vi "move.vi"(0 "M1 Info in":cluster{"M1 distance":dbl, "velocityM1":dbl}, 1 "M2 Info in":cluster{"M2 distance":dbl, "velocityM2":dbl}, 2 "button com":bool, 3 "max 1":dbl, 4 "max 2":dbl, 5 "handle":i32, 6 "halt":refnum<vi>, 7 "device ID":refnum<k1>, 8 "M3 Info in":cluster{"M3 distance":dbl, "velocityM3":dbl}, 9 "M3 Axis":u16(ring)=5 items=["X axis", "Y axis", "Z axis", "X axis rotation", "Y axis rotation", "Z axis rotation", "U axis", "V axis"], 10 "M1 Axis":u16(ring)=2 items=["X axis", "Y axis", "Z axis", "X axis rotation", "Y axis rotation", "Z axis rotation", "U axis", "V axis"], 11 "M2 Axis":u16(ring)=5 items=["X axis", "Y axis", "Z axis", "X axis rotation", "Y axis rotation", "Z axis rotation", "U axis", "V axis"], 12 "Invert":bool, 13 "Invert 2":bool=TRUE, 18 "Invert 3":bool=TRUE, 19 "max 3":dbl) -> ()   [LabVIEW 2012]
uses:
  <vilib>/Utility/inputDevices.llb/joystickAcquire.vi
  MicroDrive.dll
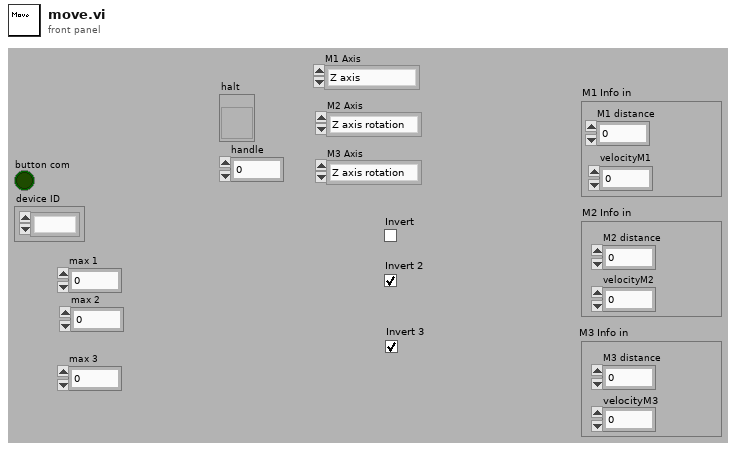
[diagram p1: front panel]
types:
  T1 = cluster{"Boolean array[0]":bool, "Boolean array[1]":bool, "Boolean array[2]":bool, "Boolean array[3]":bool, "Boolean array[4]":bool, "Boolean array[5]":bool, "Boolean array[6]":bool, "Boolean array[7]":bool, "Boolean array[8]":bool, "Boolean array[9]":bool, "Boolean array[10]":bool, "Boolean array[11]":bool, "Boolean array[12]":bool, "Boolean array[13]":bool, "Boolean array[14]":bool, "Boolean array[15]":bool}
  T2 = cluster{"X axis":i32, "Y axis":i32, "Z axis":i32, "X axis rotation":i32, "Y axis rotation":i32, "Z axis rotation":i32, "U axis":i32, "V axis":i32}
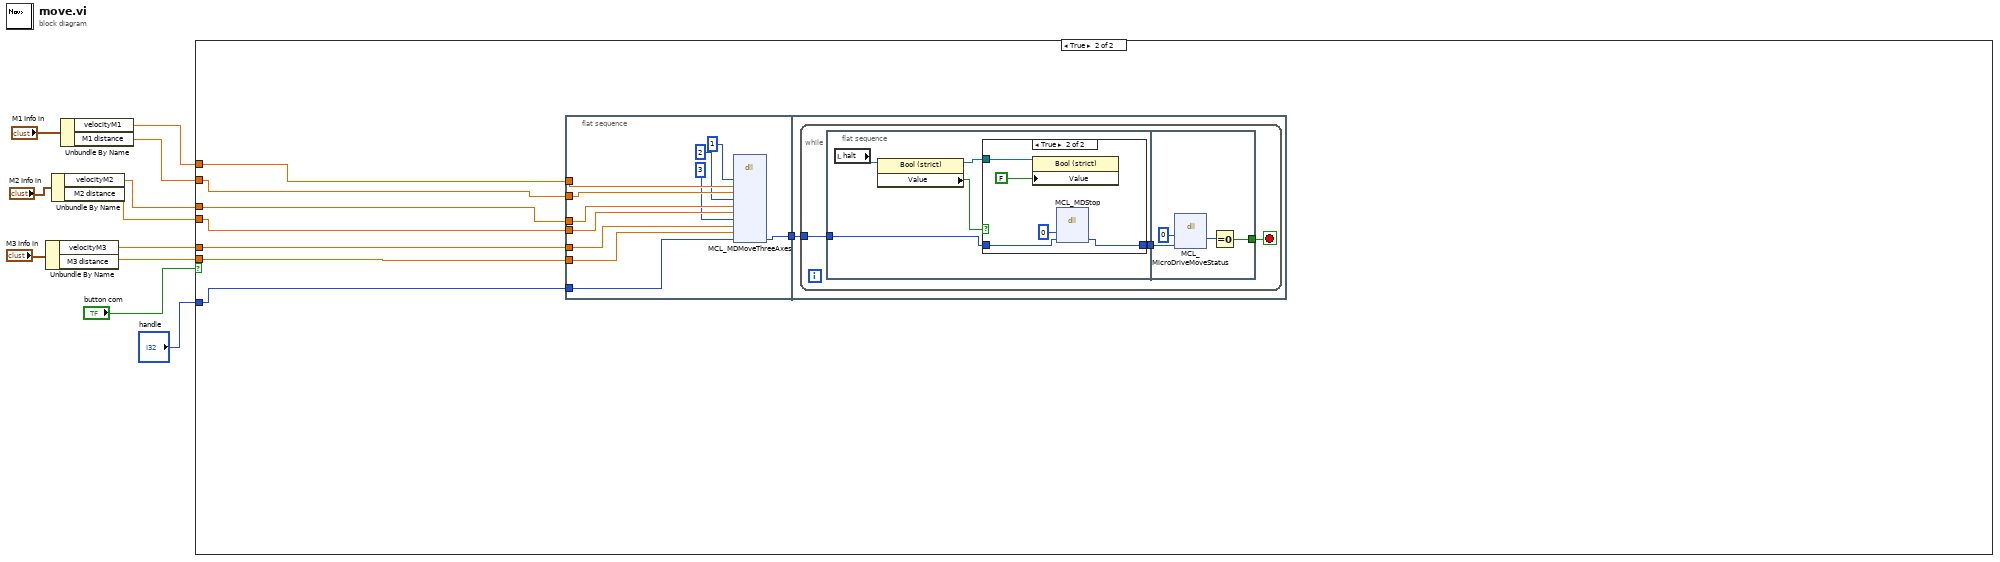
[diagram p0: block diagram]
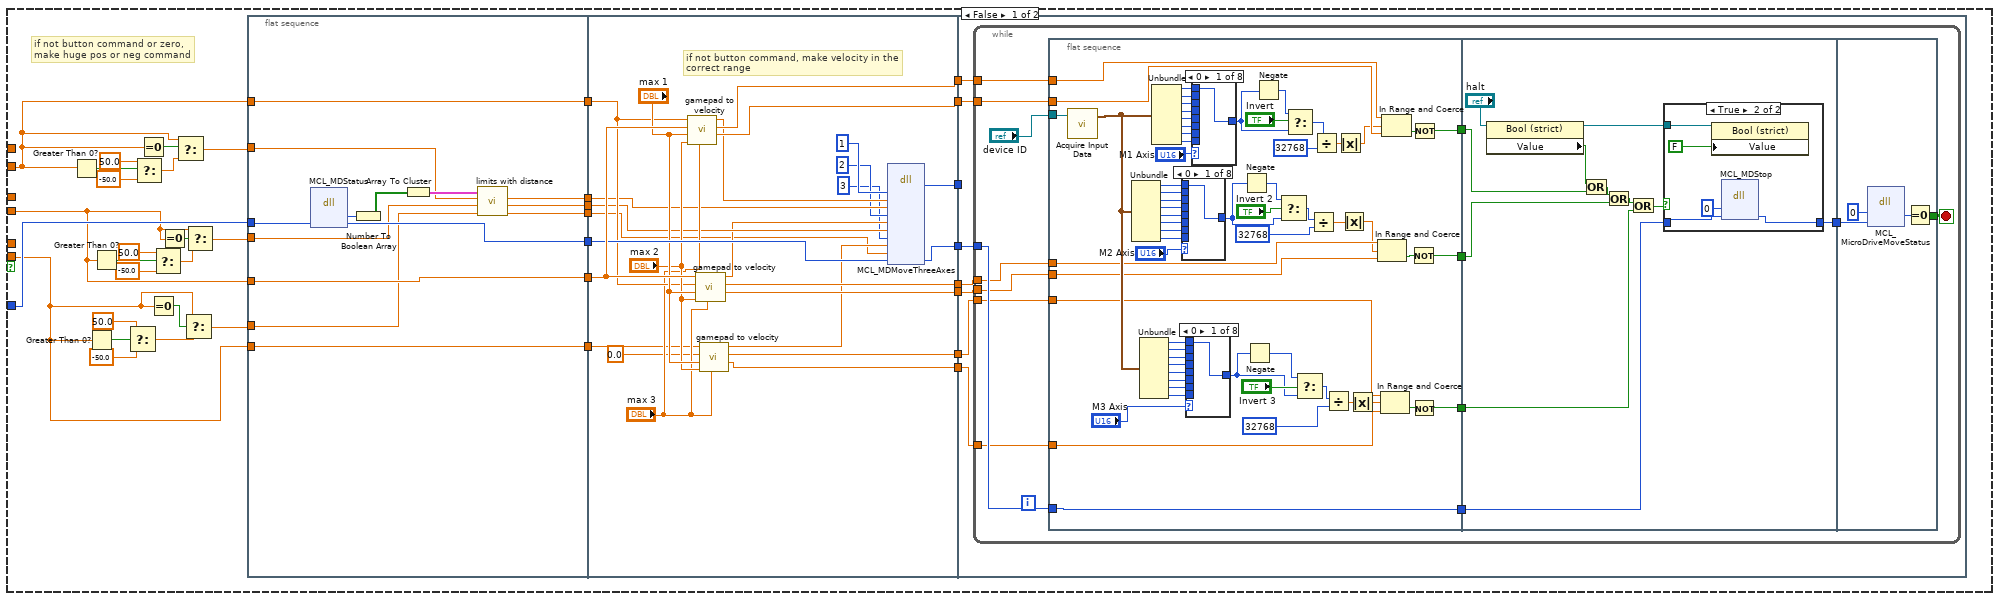
[diagram p2: hidden frame]
diagram:
  n1 = Unbundle By Name("M3 Info in") -> ("velocityM3"=w2:dbl, "M3 distance"=w1:dbl)
  n2 = Unbundle By Name("M2 Info in") -> ("velocityM2"=w4:dbl, "M2 distance"=w5:dbl)
  n3 = Unbundle By Name("M1 Info in") -> ("velocityM1"=w8:dbl, "M1 distance"=w9:dbl)
  n4 = case shown="True" "button com" {
    tunnel: "handle" -> [w29 w224]
    tunnel: w9 -> [w24 w222]
    tunnel: w8 -> [_ w221]
    tunnel: w5 -> [w20 w220]
    tunnel: w4 -> [_ w219]
    tunnel: w2 -> [_ w218]
    tunnel: w1 -> [w13 w217]
    frame False {
      # "if not button command or zero,\nmake huge pos or neg command"
      n5 = Greater Than 0?(x=w24) -> (x > 0?=w39:bool)
      n6 = Greater Than 0?(x=w13) -> (x > 0?=w19:bool)
      n7 = Greater Than 0?(x=w20) -> (x > 0?=w34:bool)
      n8 = Select(t=50.0, s=w19, f=-50.0) -> (s? t:f=w16:dbl)
      n9 = Select(t=50.0, s=w39, f=-50.0) -> (s? t:f=w40:dbl)
      n10 = Equal To 0?(x=w24) -> (x = 0?=w41:bool)
      n11 = Equal To 0?(x=w13) -> (x = 0?=w15:bool)
      n12 = Select(t=50.0, s=w34, f=-50.0) -> (s? t:f=w35:dbl)
      n13 = Equal To 0?(x=w20) -> (x = 0?=w36:bool)
      n14 = Select(t=w24, s=w41, f=w40) -> (s? t:f=w31:dbl)
      n15 = Select(t=w13, s=w15, f=w16) -> (s? t:f=w14:dbl)
      n16 = Select(t=w20, s=w36, f=w35) -> (s? t:f=w30:dbl)
      n17 = flat-sequence {
        tunnel: [w59] -> w48
        tunnel: [w52] -> w47
        tunnel: [w51] -> w46
        tunnel: [w55] -> w45
        tunnel: [w54] -> w44
        tunnel: w29 -> [w60]
        tunnel: w31 -> [w57]
        tunnel: w30 -> [w56]
        tunnel: w24 -> [w55]
        tunnel: w20 -> [w54]
        tunnel: w13 -> [w53]
        tunnel: [w53] -> w21
        tunnel: w14 -> [w50]
        tunnel: [w49] -> w12
        tunnel: [w87] -> w43
        tunnel: w48 -> [w80]
        tunnel: w47 -> [w74]
        tunnel: w46 -> [w73]
        tunnel: w45 -> [w76]
        tunnel: w44 -> [w81]
        tunnel: [w86] -> w42
        tunnel: [w85] -> w28
        tunnel: [w84] -> w27
        tunnel: [w83] -> w26
        tunnel: [w82] -> w25
        tunnel: [w72] -> w23
        tunnel: [w79] -> w22
        tunnel: w21 -> [w70]
        tunnel: w12 -> [w63]
        tunnel: w43 -> [w94]
        tunnel: w42 -> [_]
        tunnel: w28 -> [w93]
        tunnel: w27 -> [w92]
        tunnel: w26 -> [w91]
        tunnel: w25 -> [w90]
        tunnel: w23 -> [w89]
        tunnel: w22 -> [w88]
        frame #0 {
          n18 = dll-call lib="C:/Users/Labview/Desktop/SRR/MicroDrive_x64/Labview Examples/MicroDrive.dll" fn="MCL_MDStatus"("handle"=w60) -> ("status"=w62:u16, "handle"=w59:i32)  [unwired: 3 in, 4 out]
          n19 = Number To Boolean Array(number=w62) -> (Boolean array=w61:bool[])
          n20 = Array To Cluster(array=w61) -> (cluster=w58:T1)
          n21 = call "limits with distance.vi"("distanceM3"=w50, "distanceM2"=w56, "distanceM1"=w57, "cluster"=w58) -> ("M3 Distance"=w49:dbl, "M2 Distance"=w51:dbl, "M1 Distance"=w52:dbl)  [unwired: 5 out]
        }
        frame #1 {
          # "if not button command, make velocity in the\ncorrect range"
          n22 = call "gamepad to velocity.vi"("max 3 axis"="max 3", "max 2 axis"="max 2", "max 1 axis"="max 1", "joystick sub"=w81, "joystick main"=w76) -> ("lower bound"=w84:dbl, "upper bound"=w85:dbl, "Velocity"=w69:dbl)  [unwired: 4 out]
          n23 = call "gamepad to velocity.vi"("max 3 axis"="max 3", "max 2 axis"="max 2", "max 1 axis"="max 1", "joystick sub"=w76, "joystick main"=w81) -> ("lower bound"=w82:dbl, "upper bound"=w83:dbl, "Velocity"=w68:dbl)  [unwired: 4 out]
          n24 = call "gamepad to velocity.vi"("max 3 axis"="max 3", "max 2 axis"="max 2", "max 1 axis"="max 1", "joystick sub"=0.0, "joystick main"=w70) -> ("lower bound"=w79:dbl, "upper bound"=w72:dbl, "Velocity"=w67:dbl)  [unwired: 4 out]
          n25 = dll-call lib="C:/Users/Labview/Desktop/SRR/MicroDrive_x64/Labview Examples/MicroDrive.dll" fn="MCL_MDMoveThreeAxes"("axis1"=1 ("roundingX"), "velocity1"=w69, "distance1"=w74, "axis2"=2 ("roundingX"), "velocity2"=w68, "distance2"=w73, "axis3"=3 ("roundingX"), "velocity3"=w67, "distance3"=w63, "handle"=w80) -> ("return type"=w86:i32, "handle"=w87:i32)  [unwired: 11 in, 3 out]
        }
        frame #2 {
          n26 = while {
            tunnel: w94 -> [w108]
            tunnel: w93 -> [w104]
            tunnel: w92 -> [w103]
            tunnel: w91 -> [w102]
            tunnel: w90 -> [w101]
            tunnel: w89 -> [w97]
            tunnel: w88 -> [w96]
            stop <- w107 stop-if-true
            n27 = flat-sequence {
              tunnel: w108 -> [w171]
              tunnel: [w171] -> w100
              tunnel: "device ID" -> [w154]
              tunnel: w104 -> [w121]
              tunnel: w103 -> [w120]
              tunnel: w102 -> [w118]
              tunnel: w101 -> [w119]
              tunnel: [w141] -> w99
              tunnel: [w152] -> w98
              tunnel: w97 -> [w125]
              tunnel: w96 -> [w124]
              tunnel: [w122] -> w95
              tunnel: [w204] -> w106
              tunnel: w100 -> [w205]
              tunnel: w99 -> [w196]
              tunnel: w98 -> [w198]
              tunnel: w95 -> [w197]
              tunnel: [w214] -> w107
              tunnel: w106 -> [w215]
              frame #0 {
                n28 = call-poly <vilib>:"Acquire Input Data.vi"("device ID"=w154) -> ("axis info"=w138:T2)  [unwired: 2 in, 16 out]
                n29 = Unbundle(w138) -> ("X axis"=w144:i32, "Y axis"=w145:i32, "Z axis"=w146:i32, "X axis rotation"=w147:i32, "Y axis rotation"=w148:i32, "Z axis rotation"=w149:i32, "U axis"=w150:i32, "V axis"=w151:i32)
                n30 = Unbundle(w138) -> ("X axis"=w139:i32, "Y axis"=w137:i32, "Z axis"=w136:i32, "X axis rotation"=w135:i32, "Y axis rotation"=w134:i32, "Z axis rotation"=w133:i32, "U axis"=w132:i32, "V axis"=w131:i32)
                n31 = Unbundle(w138) -> ("X axis"=w156:i32, "Y axis"=w157:i32, "Z axis"=w158:i32, "X axis rotation"=w159:i32, "Y axis rotation"=w160:i32, "Z axis rotation"=w161:i32, "U axis"=w162:i32, "V axis"=w163:i32)
                n32 = case shown="0" "M2 Axis" {
                  tunnel: w144 -> [w180 _ _ _ _ _ _ _]
                  tunnel: w145 -> [_ w181 _ _ _ _ _ _]
                  tunnel: w146 -> [_ _ w182 _ _ _ _ _]
                  tunnel: w147 -> [_ _ _ w183 _ _ _ _]
                  tunnel: w148 -> [_ _ _ _ w184 _ _ _]
                  tunnel: w149 -> [_ _ _ _ _ w185 _ _]
                  tunnel: w150 -> [_ _ _ _ _ _ w186 _]
                  tunnel: w151 -> [_ _ _ _ _ _ _ w187]
                  tunnel: [w180 w181 w182 w183 w184 w185 w186 w187] -> w114
                  frame 0 {
                  }
                  frame 1 {
                  }
                  frame 2, Default {
                  }
                  frame 3 {
                  }
                  frame 4 {
                  }
                  frame 5 {
                  }
                  frame 6 {
                  }
                  frame 7 {
                  }
                }
                n33 = case shown="0" "M3 Axis" {
                  tunnel: w139 -> [w172 _ _ _ _ _ _ _]
                  tunnel: w137 -> [_ w173 _ _ _ _ _ _]
                  tunnel: w136 -> [_ _ w174 _ _ _ _ _]
                  tunnel: w135 -> [_ _ _ w175 _ _ _ _]
                  tunnel: w134 -> [_ _ _ _ w176 _ _ _]
                  tunnel: w133 -> [_ _ _ _ _ w177 _ _]
                  tunnel: w132 -> [_ _ _ _ _ _ w178 _]
                  tunnel: w131 -> [_ _ _ _ _ _ _ w179]
                  tunnel: [w172 w173 w174 w175 w176 w177 w178 w179] -> w113
                  frame 0 {
                  }
                  frame 1 {
                  }
                  frame 2, Default {
                  }
                  frame 3 {
                  }
                  frame 4 {
                  }
                  frame 5 {
                  }
                  frame 6 {
                  }
                  frame 7 {
                  }
                }
                n34 = case shown="0" "M1 Axis" {
                  tunnel: w156 -> [w188 _ _ _ _ _ _ _]
                  tunnel: w157 -> [_ w189 _ _ _ _ _ _]
                  tunnel: w158 -> [_ _ w190 _ _ _ _ _]
                  tunnel: w159 -> [_ _ _ w191 _ _ _ _]
                  tunnel: w160 -> [_ _ _ _ w192 _ _ _]
                  tunnel: w161 -> [_ _ _ _ _ w193 _ _]
                  tunnel: w162 -> [_ _ _ _ _ _ w194 _]
                  tunnel: w163 -> [_ _ _ _ _ _ _ w195]
                  tunnel: [w188 w189 w190 w191 w192 w193 w194 w195] -> w112
                  frame 0 {
                  }
                  frame 1 {
                  }
                  frame 2, Default {
                  }
                  frame 3 {
                  }
                  frame 4 {
                  }
                  frame 5 {
                  }
                  frame 6 {
                  }
                  frame 7 {
                  }
                }
                n35 = Negate(x=w114) -> (-x=w166:i32)
                n36 = Negate(x=w113) -> (-x=w129:i32)
                n37 = Negate(x=w112) -> (-x=w168:i32)
                n38 = Select(t=w166, s="Invert 2", f=w114) -> (s? t:f=w170:i32)
                n39 = Select(t=w168, s="Invert", f=w112) -> (s? t:f=w169:i32)
                n40 = Select(t=w129, s="Invert 3", f=w113) -> (s? t:f=w128:i32)
                n41 = Divide(x=w170, y=32768) -> (x/y=w153:dbl)
                n42 = Divide(x=w169, y=32768) -> (x/y=w143:dbl)
                n43 = Divide(x=w128, y=32768) -> (x/y=w126:dbl)
                n44 = Absolute Value(x=w143) -> (abs(x)=w117:dbl)
                n45 = Absolute Value(x=w153) -> (abs(x)=w116:dbl)
                n46 = Absolute Value(x=w126) -> (abs(x)=w115:dbl)
                n47 = In Range and Coerce(upper limit=w118, x=w116, lower limit=w119) -> (In Range?=w142:bool)  [unwired: 1 out]
                n48 = In Range and Coerce(upper limit=w125, x=w115, lower limit=w124) -> (In Range?=w123:bool)  [unwired: 1 out]
                n49 = In Range and Coerce(upper limit=w121, x=w117, lower limit=w120) -> (In Range?=w140:bool)  [unwired: 1 out]
                n50 = Not(x=w142) -> (.not. x?=w141:bool)
                n51 = Not(x=w123) -> (.not. x?=w122:bool)
                n52 = Not(x=w140) -> (.not. x?=w152:bool)
              }
              frame #1 {
                n53 = property on="Property Node" class="Bool (strict)"(reference="halt") -> (reference out=w203:refnum<vi>, "Value"=w202:bool)  [unwired: 1 in, 1 out]
                n54 = Or(x=w202, y=w198) -> (x .or. y?=w201:bool)
                n55 = Or(x=w201, y=w196) -> (x .or. y?=w199:bool)
                n56 = Or(x=w199, y=w197) -> (x .or. y?=w200:bool)
                n57 = case shown="True" w200 {
                  tunnel: w205 -> [w207 w210]
                  tunnel: [w207 w208] -> w204
                  tunnel: w203 -> [_ w211]
                  frame False {
                  }
                  frame True {
                    n58 = property on="Property Node" class="Bool (strict)"(reference=w211, "Value"=FALSE) -> ()  [unwired: 1 in, 2 out]
                    n59 = dll-call lib="C:/Users/Labview/Desktop/SRR/MicroDrive_x64/Labview Examples/MicroDrive.dll" fn="MCL_MDStop"("status"=u16 0, "handle"=w210) -> ("handle"=w208:i32)  [unwired: 3 in, 4 out]
                  }
                }
              }
              frame #2 {
                n60 = dll-call lib="C:/Users/Labview/Desktop/SRR/MicroDrive_x64/Labview Examples/MicroDrive.dll" fn="MCL_MicroDriveMoveStatus"("isMoving"=0 ("axis"), "handle"=w215) -> ("isMoving"=w213:i32)  [unwired: 4 in, 3 out]
                n61 = Equal To 0?(x=w213) -> (x = 0?=w214:bool)
              }
            }
          }
        }
      }
    }
    frame True {
      n62 = flat-sequence {
        tunnel: w222 -> [w230]
        tunnel: w220 -> [w229]
        tunnel: w221 -> [w235]
        tunnel: w224 -> [w234]
        tunnel: w219 -> [w233]
        tunnel: [w232] -> w223
        tunnel: w218 -> [w231]
        tunnel: w217 -> [w228]
        tunnel: w223 -> [w236]
        frame #0 {
          n63 = dll-call lib="C:/Users/Labview/Desktop/SRR/MicroDrive_x64/Labview Examples/MicroDrive.dll" fn="MCL_MDMoveThreeAxes"("axis1"=1 ("roundingX"), "velocity1"=w235, "distance1"=w230, "axis2"=2 ("roundingX"), "velocity2"=w233, "distance2"=w229, "axis3"=3 ("roundingX"), "velocity3"=w231, "distance3"=w228, "handle"=w234) -> ("handle"=w232:i32)  [unwired: 11 in, 4 out]
        }
        frame #1 {
          n64 = while {
            tunnel: w236 -> [w239]
            stop <- w237 stop-if-true
            n65 = flat-sequence {
              tunnel: w239 -> [w242]
              tunnel: [w240] -> w238
              tunnel: w238 -> [w252]
              tunnel: [w251] -> w237
              frame #0 {
                n66 = local read "halt"() -> (w241:refnum<vi>)
                n67 = property on="Property Node" class="Bool (strict)"(reference=w241) -> (reference out=w244:refnum<vi>, "Value"=w243:bool)  [unwired: 1 in, 1 out]
                n68 = case shown="True" w243 {
                  tunnel: w242 -> [w245 w246]
                  tunnel: [w245 w247] -> w240
                  tunnel: w244 -> [_ w249]
                  frame False {
                  }
                  frame True {
                    n69 = property on="Property Node" class="Bool (strict)"(reference=w249, "Value"=FALSE) -> ()  [unwired: 1 in, 2 out]
                    n70 = dll-call lib="C:/Users/Labview/Desktop/SRR/MicroDrive_x64/Labview Examples/MicroDrive.dll" fn="MCL_MDStop"("status"=u16 0, "handle"=w246) -> ("handle"=w247:i32)  [unwired: 3 in, 4 out]
                  }
                }
              }
              frame #1 {
                n71 = dll-call lib="C:/Users/Labview/Desktop/SRR/MicroDrive_x64/Labview Examples/MicroDrive.dll" fn="MCL_MicroDriveMoveStatus"("isMoving"=u32 0 ("axis"), "handle"=w252) -> ("isMoving"=w253:i32)  [unwired: 4 in, 3 out]
                n72 = Equal To 0?(x=w253) -> (x = 0?=w251:bool)
              }
            }
          }
        }
      }
    }
  }
